vi "WriteRecMsg2List.vi"(9 "tsapp_receive_can_messageList":T1[](array[typedef]), 11 "Table输入":refnum<vi>) -> ()   [LabVIEW 2016]
uses:
  MessageInfo.ctl
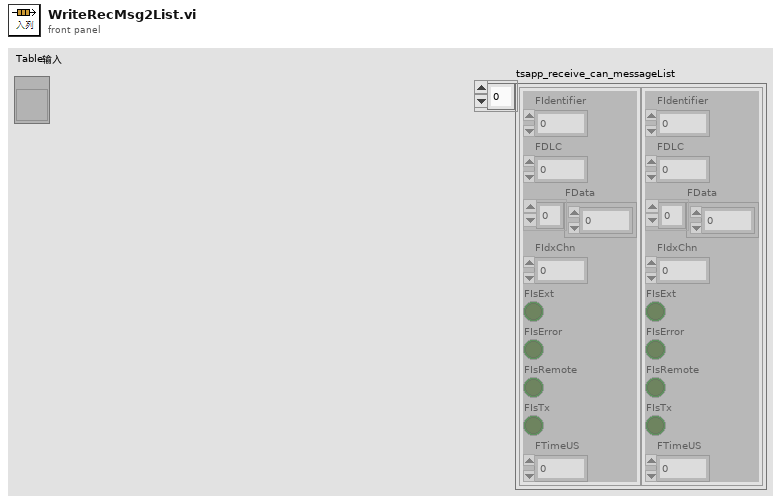
[diagram p1: front panel]
types:
  T1 = typedef "MessageInfo.ctl" = cluster{"FIdentifier":i32, "FDLC":u8, "FData":u8[], "FIdxChn":u8, "FIsExt":bool, "FIsError":bool, "FIsRemote":bool, "FIsTx":bool, "FTimeUS":u64}
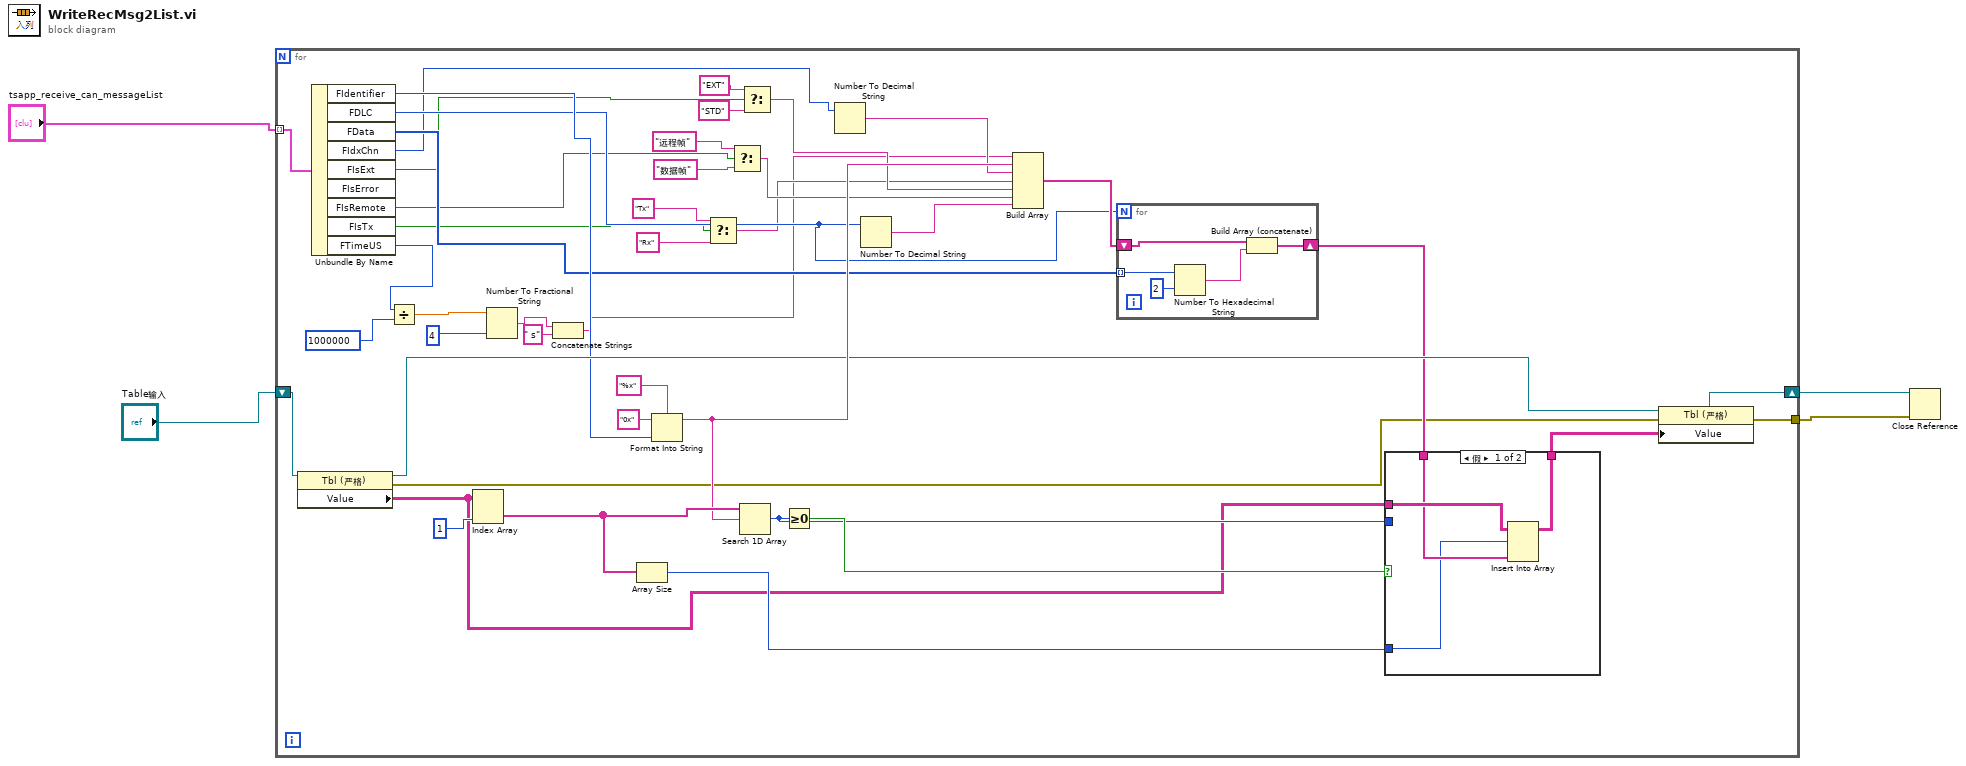
[diagram p0: block diagram]
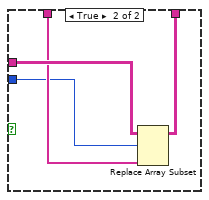
[diagram p2: hidden frame]
diagram:
  n1 = for {
    tunnel: [w33] -> w2
    shift-right: [w34] -> w3
    shift-left: "Table输入" -> [w44]
    tunnel: "tsapp_receive_can_messageList" -> [w28] mode=indexing
    n2 = property class="Tbl (严格)"(reference=w44) -> (reference out=w35:refnum<vi>, error out=w29:errorcluster, "Value"=w32:string[][])  [unwired: 1 in]
    n3 = Unbundle By Name(w28) -> ("FIdentifier"=w27:i32, "FDLC"=w26:u8, "FData"=w25:u8[], "FIdxChn"=w23:u8, "FIsExt"=w24:bool, "FIsRemote"=w18:bool, "FIsTx"=w15:bool, "FTimeUS"=w10:u64)  [unwired: 1 out]
    n4 = Divide(x=w10, y=1000000) -> (x/y=w9:dbl)
    n5 = Index Array(array=w32, index (col)=1 ("禁用的索引 (列)")) -> (element=w41:string[])  [unwired: 1 in]
    n6 = Number To Fractional String(number=w9, precision (6)=i16 4 ("精度(6)")) -> (F-format string=w7:string)  [unwired: 2 in]
    n7 = Concatenate Strings(w7, " s" ("字符串")) -> (w6:string)
    n8 = Array Size(array=w41) -> (size(s)=w40:i32)
    n9 = Format Into String(format string="%x" ("格式字符串"), initial string="0x" ("初始字符串"), w27) -> (resulting string=w39:string)  [unwired: 1 in, 1 out]
    n10 = Select(t="Tx", s=w15, f="Rx") -> (s? t:f=w14:string)
    n11 = Select(t="远程帧", s=w18, f="数据帧") -> (s? t:f=w19:string)
    n12 = Search 1D Array(1D array=w41, element=w39) -> (index of element=w42:i32)  [unwired: 1 in]
    n13 = Select(t="EXT", s=w24, f="STD") -> (s? t:f=w20:string)
    n14 = Greater Or Equal To 0?(x=w42) -> (x >= 0?=w43:bool)
    n15 = Number To Decimal String(number=w23) -> (decimal integer string=w38:string)  [unwired: 1 in]
    n16 = Number To Decimal String(number=w26) -> (decimal integer string=w37:string)  [unwired: 1 in]
    n17 = Build Array(w6, w39, w38, w14, w20, w19, w37) -> (w36:string[])
    n18 = for {
      N: w26 -> [_]
      tunnel: w25 -> [w52] mode=indexing
      shift-right: [w49] -> w31
      shift-left: w36 -> [w48]
      n19 = Number To Hexadecimal String(1:i16 2 ("宽度(-)"), 2:w52) -> (0:w50:string)
      n20 = Build Array (concatenate)(w48, w50) -> (w49:string[])
    }
    n21 = case shown="假" w43 {
      tunnel: w42 -> [_ w58]
      tunnel: w40 -> [w54 _]
      tunnel: w32 -> [w56 w60]
      tunnel: w31 -> [w55 w59]
      tunnel: [w53 w57] -> w30
      frame False {
        n22 = Insert Into Array(array=w56, index (row)=w54, new element=w55) -> (w53:string[][])  [unwired: 1 in]
      }
      frame True {
        n23 = Replace Array Subset(array=w60, new element=w59, index (row)=w58) -> (w57:string[][])  [unwired: 1 in]
      }
    }
    n24 = property class="Tbl (严格)"(reference=w35, error in=w29, "Value"=w30) -> (reference out=w34:refnum<vi>, error out=w33:errorcluster)
  }
  n25 = Close Reference(reference=w3, error in (no error)=w2) -> ()  [unwired: 1 out]
